vi "XBox-Vibrate.vi"(0 "Left Motor":dbl, 5 "Right Motor":dbl, 7 "Duration (ms)":u32, 11 "error in (no error)":errorcluster) -> (15 "error out":errorcluster)   [LabVIEW 2015]
uses:
  Microsoft.Xna.Framework
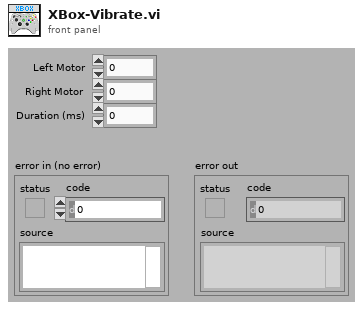
[diagram p1: front panel]
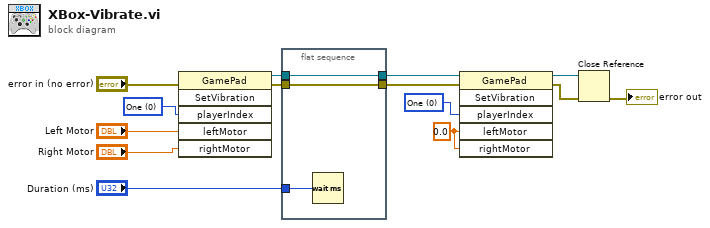
[diagram p0: block diagram]
diagram:
  w4 = sgl 0.0 ("leftMotor")
  w5 = 0 items=["One", "Two", "Three", "Four"] ("playerIndex")
  w14 = 0 items=["One", "Two", "Three", "Four"] ("playerIndex")
  n1 = invoke class="GamePad" method="SetVibration"(error in="error in (no error)", "playerIndex"=w14, "leftMotor"="Left Motor", "rightMotor"="Right Motor") -> (reference out=w10:refnum<k24>, error out=w9:errorcluster)  [unwired: 2 in, 4 out]
  n2 = flat-sequence {
    tunnel: w10 -> [w16]
    tunnel: w9 -> [w15]
    tunnel: "Duration (ms)" -> [w17]
    tunnel: [w16] -> w7
    tunnel: [w15] -> w6
    frame #0 {
      n3 = Wait (ms)(milliseconds to wait=w17) -> ()  [unwired: 1 out]
    }
  }
  n4 = invoke class="GamePad" method="SetVibration"(reference=w7, error in=w6, "playerIndex"=w5, "leftMotor"=w4, "rightMotor"=w4) -> (reference out=w2:refnum<k24>, error out=w3:errorcluster)  [unwired: 1 in, 4 out]
  n5 = Close Reference(reference=w2, error in (no error)=w3) -> (error out=→"error out":errorcluster)
